vi "SetCursorPos.vi"(1 "dy":i32, 2 "dx":i32) -> ()   [LabVIEW 2018]
uses:
  User32.dll
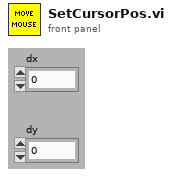
[diagram p1: front panel]
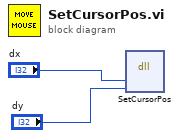
[diagram p0: block diagram]
diagram:
  n1 = dll-call lib="User32.dll" fn="SetCursorPos"("dx"="dx", "dy"="dy") -> ()  [unwired: 6 in, 2 out]
